vi "get_component_type_name.vi"(8 "error in (no error)":errorcluster, 11 "GenericDataCollection in":refnum<class "GenericDataCollection.lvclass">) -> (0 "error out":errorcluster, 2 "component type":string="DataCollection", 3 "GenericDataCollection out":refnum<class "GenericDataCollection.lvclass">)   [LabVIEW 2010, in "GenericDataCollection.lvclass"]
uses:
  GenericDataCollection.lvclass
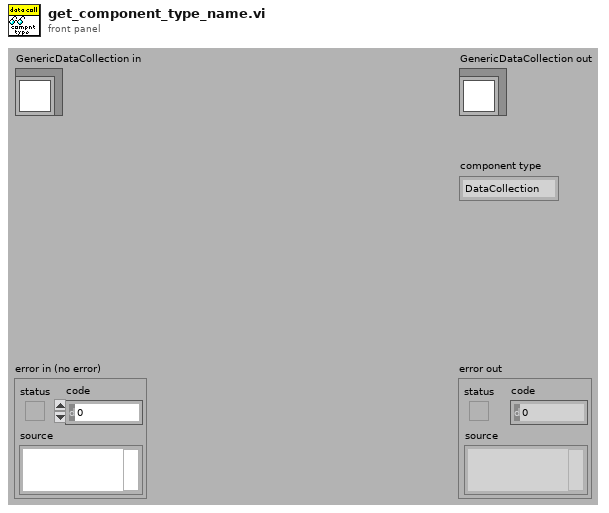
[diagram p1: front panel]
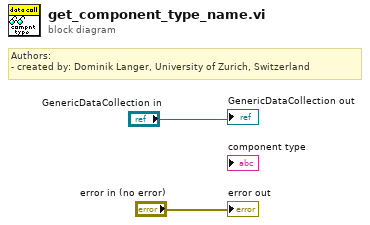
[diagram p0: block diagram]
diagram:
  # "Authors: \n- created by: Dominik Langer, University of Zurich, Switzerland"
  "error out" <- "error in (no error)"
  "GenericDataCollection out" <- "GenericDataCollection in"
